vi "GenerateAPIEvent_Motor Controller.vi"(6 "Timeout (ms)":u32=600000, 7 "Wait (F)":bool, 8 "error in (no error)":errorcluster, 9 "Task ID":string, 10 "API Command Cluster":T1, 11 "Motor Controller In":refnum<class "Motor Controller.lvclass">) -> (0 "error out":errorcluster, 2 "Return Value":variant, 3 "Motor Controller out":refnum<class "Motor Controller.lvclass">)   [LabVIEW 2022 SP3, in "Motor Controller.lvclass"]
uses:
  Motor Controller.lvclass
  Typedefs/API Command Cluster.ctl
  Typedefs/API Command Enum.ctl
  Typedefs/API Event Data.ctl
  Typedefs/API Task State.ctl
  Motor Controller.lvclass/Motor Controller.ctl
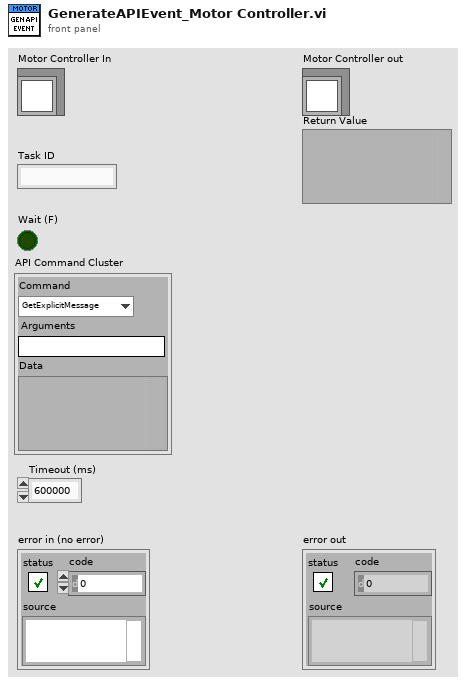
[diagram p1: front panel]
types:
  T1 = typedef "Motor Controller.lvclass/API Command Cluster.ctl" = cluster{"Command":T2, "Arguments":string, "Data":variant}
  T2 = typedef "Motor Controller.lvclass/API Command Enum.ctl" = enum16{"GetExplicitMessage", "SetExplicitMessage", "Execute Stage Move Recipe", "Read Stage Move Recipe", "Abort"}
  T3 = typedef "Motor Controller.lvclass/API Task State.ctl" = enum16{"Completed", "Errored", "Pending"}
  T4 = typedef "Motor Controller.lvclass/API Event Data.ctl" = cluster{"Task":cluster{"Time Stamp":timestamp, "Timeout (ms)":u32, "Task State":T3, "Task Error":errorcluster, "Task ID":string}, "Command":variant, "Return Value":variant}
  T5 = typedef "Motor Controller.lvclass/Private Data.ctl" = cluster{"UserEvents":T6, "All Dependencies":cluster{"Class References":refnum<class>[], "Class Names":string[]}, "Status":T7}
  T6 = typedef "Motor Controller.lvclass/UserEvents.ctl" = cluster{"API Incoming Event":refnum<user-event>, "API Executed Event":refnum<user-event>, "API Return Event":refnum<user-event>, "Status Changed Event":refnum<user-event>, "StopEvent":refnum<user-event>}
  T7 = typedef "Motor Controller.lvclass/Status.ctl" = cluster{"Motor Controller Config Data":T8, "Motor Controller Data":cluster{"Enabled?":bool}, "Stage Move":T9, "Stage Busy?":bool}
  T8 = typedef "Motor Controller.lvclass/Motor Controller Config Data.ctl" = cluster{"Motor IP Addresss":string, "Current Position":i32, "Pulse_Per_mm":i32, "PrePrint":dbl[], "Load Position_mm":i32, "Laminate Position_mm":i32}
  T9 = typedef "Motor Controller.lvclass/Stage Move Data.ctl" = cluster{"Current Step":string, "Move Data":T10[]}
  T10 = typedef "Motor Controller.lvclass/Batch Index Speed Data.ctl" = cluster{"Batch & Cycle":string, "Move":cluster{"Index_mm":i32, "Speed_mm_s":i32}, "Status":T11}
  T11 = typedef "Motor Controller.lvclass/Move Status.ctl" = enum16{"Pending", "In Progress", "Completed"}
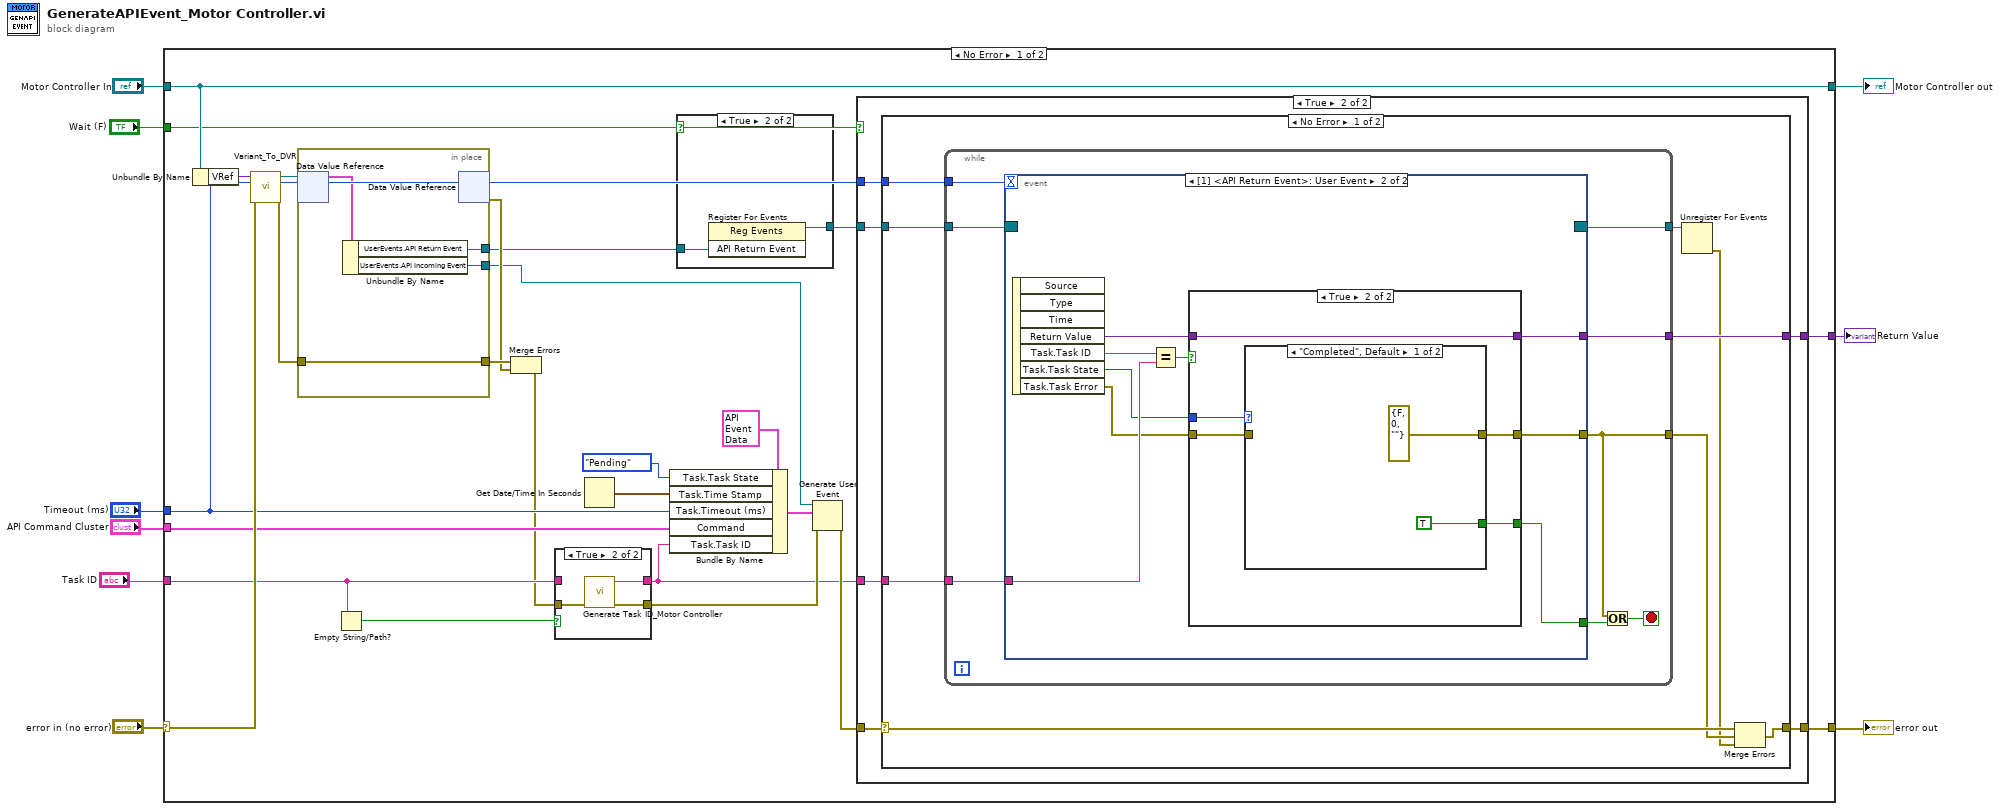
[diagram p0: block diagram]
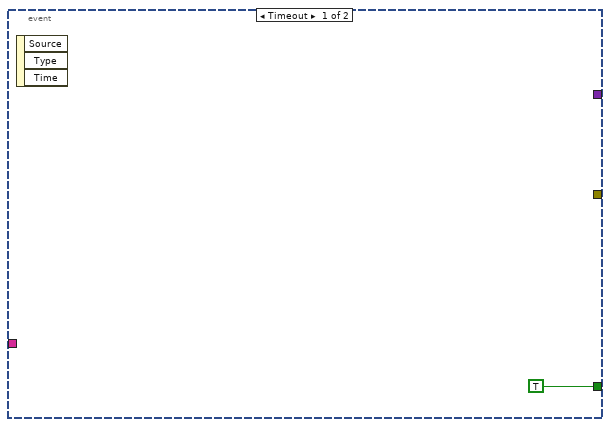
[diagram p4: hidden frame]
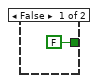
[diagram p5: hidden frame]
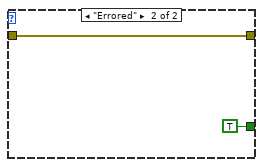
[diagram p6: hidden frame]
diagram:
  n1 = case shown="No Error" "error in (no error)" {
    selector: "error in (no error)" -> [w34 w92]
    tunnel: [w15 w92] -> w8
    tunnel: [w28 w91] -> w6
    tunnel: "Motor Controller In" -> [w28 w91]
    tunnel: "Wait (F)" -> [w21 _]
    tunnel: "Timeout (ms)" -> [w19 _]
    tunnel: "API Command Cluster" -> [w22 _]
    tunnel: [w16 _] -> w2
    tunnel: "Task ID" -> [w13 _]
    frame No Error {
      n2 = Unbundle By Name(w28) -> ("VRef"=w33:variant)
      n3 = call "Variant_To_DVR.vi"("error in (no error)"=w34, "Variant"=w33) -> ("error out"=w31:errorcluster, "DVR"=w32:refnum<data-value>)  [unwired: 8 in]
      n4 = in-place {
        in-place-border: w31 -> [w89]
        in-place-border: [w89] -> w30
        in-place-border: [w88] -> w27
        in-place-border: [w87] -> w26
        n5 = in-place-dvr #1(w32) -> (w90:T5)  [unwired: 1 out]
        n6 = Unbundle By Name(w90) -> ("UserEvents.API Return Event"=w88:refnum<user-event>, "UserEvents.API Incoming Event"=w87:refnum<user-event>)
        n7 = in-place-dvr #1() -> (w29:errorcluster)  [unwired: 1 in, 1 out]
      }
      n8 = Empty String/Path?(string/path=w13) -> (empty?=w14:bool)
      n9 = Merge Errors(w30, w29) -> (w12:errorcluster)
      n10 = case shown="True" w14 {
        tunnel: [w36 w39] -> w10
        tunnel: w13 -> [w36 _]
        tunnel: w12 -> [w35 w38]
        tunnel: [w35 w37] -> w11
        frame False {
        }
        frame True {
          n11 = call "Generate Task ID_Motor Controller.vi"("error in (no error)"=w38) -> ("error out"=w37:errorcluster, "Task ID"=w39:string)  [unwired: 9 in]
        }
      }
      n12 = Get Date/Time In Seconds() -> (seconds since 1Jan1904=w24:timestamp)
      n13 = Bundle By Name(cluster=T4 {"Task"={"Time Stamp"=timestamp(0 s since 1904-01-01), "Timeout (ms)"=0, "Task State"=enum."Completed", "Task Error"={"status"=FALSE, "code"=0, "source"=""}, "Task ID"=""}, "Command"=variant, "Return Value"=variant} ("event data"), "Task.Task State"=API_Task_State."Pending", "Task.Time Stamp"=w24, "Task.Timeout (ms)"=w19, "Command"=w22, "Task.Task ID"=w10) -> (w23:T4)
      n14 = case shown="True" w21 {
        tunnel: w27 -> [_ w86]
        tunnel: [_ w85] -> w18
        frame False {
        }
        frame True {
          n15 = register-events(w86) -> (reference out=w85:refnum<event-registration>)  [unwired: 2 in, 1 out]
        }
      }
      n16 = Generate User Event(user event=w26, event data cluster=w23, error in=w11) -> (error out=w20:errorcluster)  [unwired: 1 in, 1 out]
      n17 = case shown="True" w21 {
        tunnel: w20 -> [w40 w46]
        tunnel: w19 -> [_ w45]
        tunnel: w18 -> [_ w44]
        tunnel: [_ w43] -> w16
        tunnel: [w40 w42] -> w15
        tunnel: w10 -> [_ w41]
        frame False {
        }
        frame True {
          n18 = case shown="No Error" w46 {
            selector: w46 -> [w51 w84]
            tunnel: w45 -> [w55 _]
            tunnel: w44 -> [w54 _]
            tunnel: [w53 _] -> w43
            tunnel: [w48 w84] -> w42
            tunnel: w41 -> [w47 _]
            frame No Error {
              n19 = while {
                tunnel: w55 -> [w63]
                tunnel: w54 -> [w62]
                tunnel: [w61] -> w53
                tunnel: [w58] -> w52
                tunnel: [w57] -> w50
                tunnel: w47 -> [w56]
                stop <- w59 stop-if-true
                n20 = event shown="[1] <API Return Event>: User Event" {
                  selector: w62 -> [_ _]
                  dyn-events: [_ _] -> w58
                  timeout: w63 -> [_ _]
                  tunnel: [_ w69] -> w61
                  tunnel: [_ w68] -> w57
                  tunnel: [TRUE w65] -> w60
                  tunnel: w56 -> [_ w72]
                  event Timeout {
                    n21 = event-data() -> ()  [unwired: 1 in, 3 out]
                  }
                  event User Event {
                    n22 = event-data() -> ("Return Value"=w71:variant, "Task.Task ID"=w73:string, "Task.Task State"=w67:T3, "Task.Task Error"=w66:errorcluster)  [unwired: 1 in, 3 out]
                    n23 = Equal?(x=w73, y=w72) -> (x = y?=w70:bool)
                    n24 = case shown="True" w70 {
                      tunnel: w67 -> [_ w79]
                      tunnel: w66 -> [_ w78]
                      tunnel: [_ w77] -> w69
                      tunnel: w71 -> [_ w77]
                      tunnel: [_ w76] -> w68
                      tunnel: [FALSE w75] -> w65
                      frame False {
                      }
                      frame True {
                        n25 = case shown="\"Completed\", Default" w79 {
                          tunnel: w78 -> [_ w83]
                          tunnel: [errorcluster {"status"=FALSE, "code"=0, "source"=""} ("Task Error") w83] -> w76
                          tunnel: [TRUE TRUE] -> w75
                          frame "Completed", Default {
                          }
                          frame "Errored" {
                          }
                        }
                      }
                    }
                  }
                }
                n26 = Or(x=w57, y=w60) -> (x .or. y?=w59:bool)
              }
              n27 = Unregister For Events(event registration refnum=w52) -> (error out=w49:errorcluster)  [unwired: 1 in]
              n28 = Merge Errors(w51, w50, w49) -> (w48:errorcluster)
            }
            frame Error {
            }
          }
        }
      }
    }
    frame Error {
    }
  }
  "error out" <- w8
  "Motor Controller out" <- w6
  "Return Value" <- w2
